vi "practica13RNA.vi"() -> ()   [LabVIEW 2016]
panel:
  out "Boolean":bool
  out "a":dbl
  in  "x":dbl[](array[numeric])
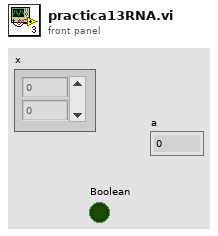
[diagram p1: front panel]
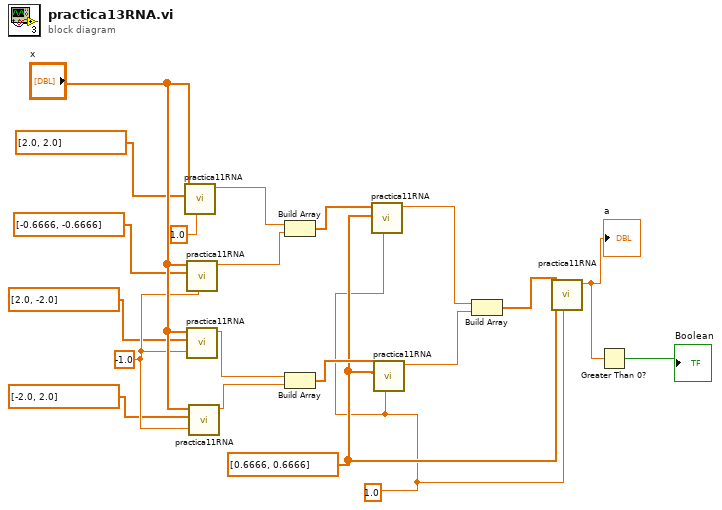
[diagram p0: block diagram]
diagram:
  w3 = 1.0 ("b")
  w4 = dbl[] [0.6666, 0.6666] ("w")
  w18 = -1.0 ("b")
  n1 = call "practica11RNA.vi"("b"=1.0, "w"=dbl[] [2.0, 2.0], "x"="x") -> ("a"=w13:dbl)  [unwired: 8 in]
  n2 = call "practica11RNA.vi"("b"=w18, "w"=dbl[] [-0.6666, -0.6666], "x"="x") -> ("a"=w12:dbl)  [unwired: 8 in]
  n3 = call "practica11RNA.vi"("b"=w18, "w"=dbl[] [2.0, -2.0], "x"="x") -> ("a"=w10:dbl)  [unwired: 8 in]
  n4 = call "practica11RNA.vi"("b"=w18, "w"=dbl[] [-2.0, 2.0], "x"="x") -> ("a"=w9:dbl)  [unwired: 8 in]
  n5 = Build Array(w13, w12) -> (w11:dbl[])
  n6 = Build Array(w10, w9) -> (w8:dbl[])
  n7 = call "practica11RNA.vi"("b"=w3, "w"=w4, "x"=w11) -> ("a"=w7:dbl)  [unwired: 8 in]
  n8 = call "practica11RNA.vi"("b"=w3, "w"=w4, "x"=w8) -> ("a"=w6:dbl)  [unwired: 8 in]
  n9 = Build Array(w7, w6) -> (w5:dbl[])
  n10 = call "practica11RNA.vi"("b"=w3, "w"=w4, "x"=w5) -> ("a"=w2:dbl)  [unwired: 8 in]
  "a" <- w2
  n11 = Greater Than 0?(x=w2) -> (x > 0?=→"Boolean":bool)
